vi "Read Controls.vi"(11 "Message Scripter in":refnum<class "Message Scripter.lvclass">) -> (1 "Wiring Rules":T1(array[ring]), 2 "Controls[]":refnum<vi>[](array[refnum]))   [LabVIEW 2020, in "Message Maker.lvlib" / "Message Scripter.lvclass"]
uses:
  Message Scripter.lvclass
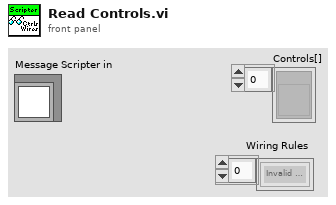
[diagram p1: front panel]
types:
  T1 = enum16{"Invalid Wire Rule", "Required", "Recommended", "Optional", "Dynamic Dispatch"}[]
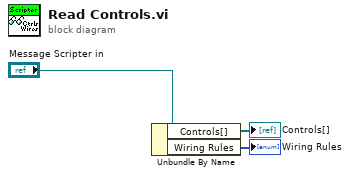
[diagram p0: block diagram]
diagram:
  n1 = Unbundle By Name("Message Scripter in") -> ("Controls[]"=→"Controls[]":refnum<vi>[], "Wiring Rules"=→"Wiring Rules":T1)
